vi "Read.vi"(4 "Error In":errorcluster, 5 "timeout ms (5000)":i32=5000, 7 "WebSocket Connection in":refnum<k5>) -> (0 "Error Out":errorcluster, 1 "Opcode":u8, 2 "Data":string, 3 "WebSocket Connection out":refnum<k5>)   [LabVIEW 2020, in "WebSockets.lvlib"]
doc: "Reads and decodes an incoming WebSockets message.\nWebSockets API 1.3.0.13\nSam Sharp - Intelligent Energy\nCopyright (c) 2015, Intelligent Energy"
uses:
  WebSockets.lvlib
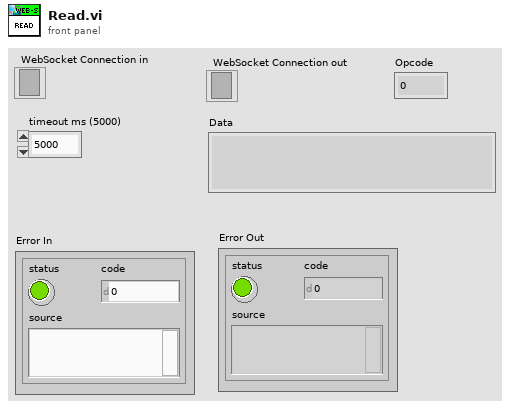
[diagram p1: front panel]
types:
  T1 = enum16{"big-endian, network order", "native, host order", "little-endian"}
  T2 = enum16{"Standard", "Buffered", "CRLF", "Immediate"}
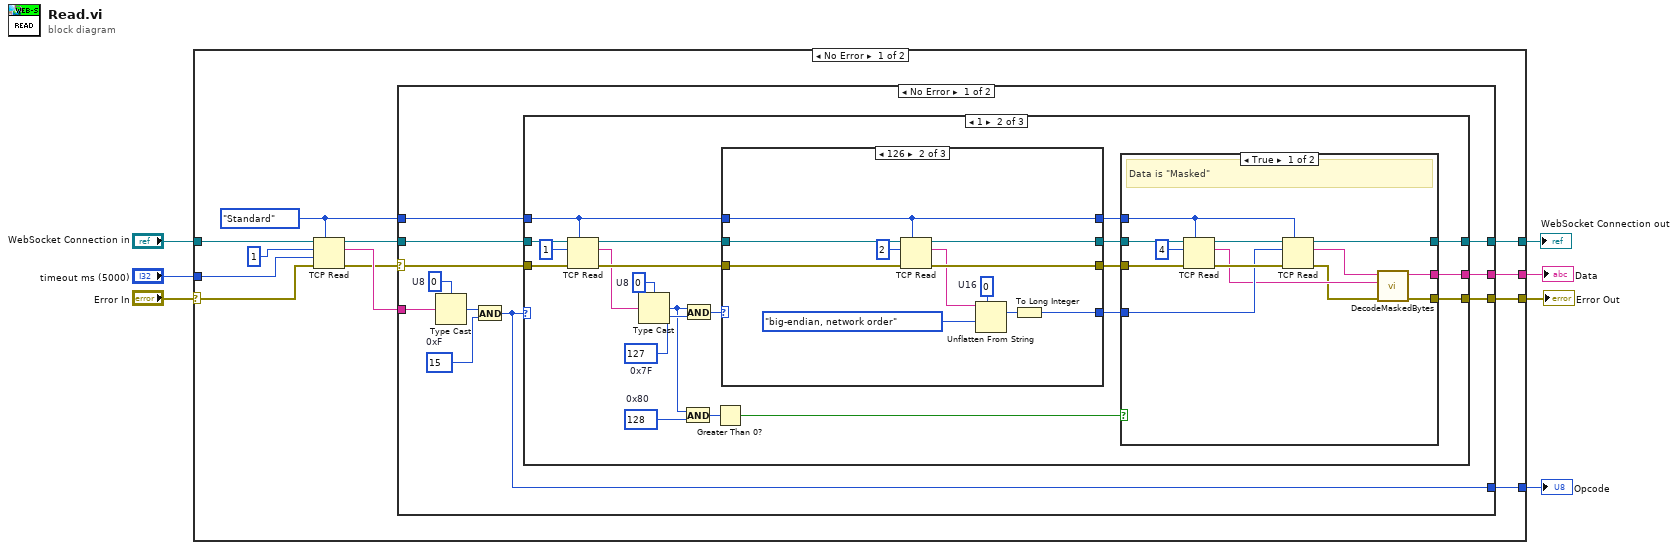
[diagram p0: block diagram]
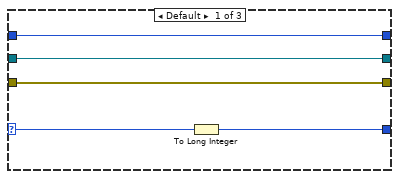
[diagram p3: hidden frame]
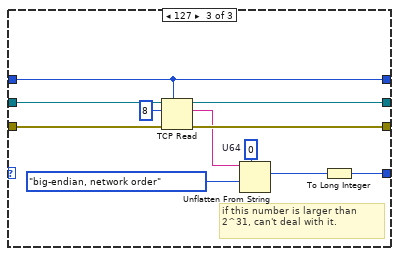
[diagram p4: hidden frame]
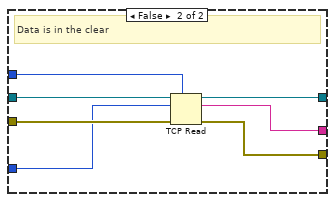
[diagram p5: hidden frame]
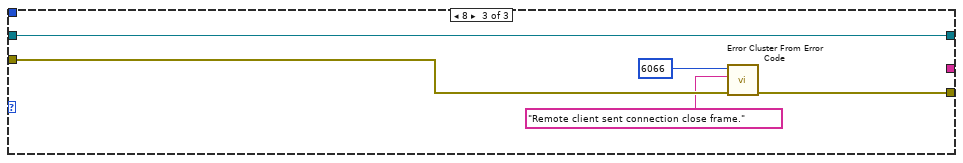
[diagram p6: hidden frame]
diagram:
  n1 = case shown="No Error" "Error In" {
    selector: "Error In" -> [w13 w109]
    tunnel: "WebSocket Connection in" -> [w19 w108]
    tunnel: [w14 w108] -> w6
    tunnel: [w12 _] -> w5
    tunnel: [w11 w109] -> w3
    tunnel: "timeout ms (5000)" -> [w10 _]
    tunnel: [w8 _] -> w1
    frame No Error {
      w15 = T2."Standard" ("mode (standard)")
      n2 = TCP Read(connection ID=w19, bytes to read=1, error in (no error)=w13, 7:w15, 9:w10) -> (connection ID out=w16:refnum<k5>, data out=w17:string, error out=w9:errorcluster)
      n3 = case shown="No Error" w9 {
        selector: w9 -> [w25 w106]
        tunnel: w17 -> [w24 _]
        tunnel: w16 -> [w30 w107]
        tunnel: w15 -> [w29 _]
        tunnel: [w28 w107] -> w14
        tunnel: [w27 _] -> w12
        tunnel: [w26 w106] -> w11
        tunnel: [w20 _] -> w8
        frame No Error {
          w21 = u8 15  # 0xF
          w23 = u8 0  # U8
          n4 = Type Cast(type=w23, x=w24) -> (*(type *) &x=w22:u8)
          n5 = And(x=w22, y=w21) -> (x .and. y?=w20:u8)
          n6 = case shown="1" w20 {
            tunnel: w30 -> [w32 w44 w105]
            tunnel: w29 -> [_ w42 _]
            tunnel: [w32 w53 w105] -> w28
            tunnel: [_ w46 _] -> w27
            tunnel: [w31 w45 w104] -> w26
            tunnel: w25 -> [w31 w40 w103]
            frame Default {
            }
            frame 1 {
              w36 = u8 128  # 0x80
              w37 = u8 0  # U8
              w52 = u8 127  # 0x7F
              n7 = TCP Read(connection ID=w44, bytes to read=1, error in (no error)=w40, 7:w42) -> (connection ID out=w43:refnum<k5>, data out=w38:string, error out=w39:errorcluster)  [unwired: 1 in]
              n8 = Type Cast(type=w37, x=w38) -> (*(type *) &x=w35:u8)
              n9 = And(x=w35, y=w36) -> (x .and. y?=w34:u8)
              n10 = And(x=w35, y=w52) -> (x .and. y?=w51:u8)
              n11 = Greater Than 0?(x=w34) -> (x > 0?=w33:bool)
              n12 = case shown="126" w51 {
                selector: w51 -> [w57 _ _]
                tunnel: w43 -> [w58 w69 w79]
                tunnel: [w58 w68 w78] -> w50
                tunnel: w42 -> [w55 w66 w74]
                tunnel: [w56 w59 w77] -> w47
                tunnel: [w55 w66 w74] -> w49
                tunnel: [w54 w65 w76] -> w48
                tunnel: w39 -> [w54 w64 w75]
                frame Default {
                  n13 = To Long Integer(number=w57) -> (32bit integer=w56:i32)
                }
                frame 126 {
                  w63 = u16 0  # U16
                  n14 = TCP Read(connection ID=w69, bytes to read=2, error in (no error)=w64, 7:w66) -> (connection ID out=w68:refnum<k5>, data out=w61:string, error out=w65:errorcluster)  [unwired: 1 in]
                  n15 = Unflatten From String(type=w63, binary string=w61, byte order (0:big-endian, network order)=T1."big-endian, network order") -> (value=w60:u16)  [unwired: 2 in, 2 out]
                  n16 = To Long Integer(number=w60) -> (32bit integer=w59:i32)
                }
                frame 127 {
                  w73 = u64 0  # U64
                  # "if this number is larger than\n2^31, can't deal with it."
                  n17 = TCP Read(connection ID=w79, bytes to read=8, error in (no error)=w75, 7:w74) -> (connection ID out=w78:refnum<k5>, data out=w72:string, error out=w76:errorcluster)  [unwired: 1 in]
                  n18 = Unflatten From String(type=w73, binary string=w72, byte order (0:big-endian, network order)=T1."big-endian, network order") -> (value=w71:u64)  [unwired: 2 in, 2 out]
                  n19 = To Long Integer(number=w71) -> (32bit integer=w77:i32)
                }
              }
              n20 = case shown="True" w33 {
                tunnel: [w93 w100] -> w53
                tunnel: w50 -> [w92 w99]
                tunnel: w49 -> [w90 w98]
                tunnel: w48 -> [w89 w97]
                tunnel: w47 -> [w86 w96]
                tunnel: [w83 w94] -> w46
                tunnel: [w81 w95] -> w45
                frame True {
                  # "Data is \"Masked\""
                  n21 = TCP Read(connection ID=w92, bytes to read=4, error in (no error)=w89, 7:w90) -> (connection ID out=w91:refnum<k5>, data out=w85:string, error out=w88:errorcluster)  [unwired: 1 in]
                  n22 = TCP Read(connection ID=w91, bytes to read=w86, error in (no error)=w88, 7:w90) -> (connection ID out=w93:refnum<k5>, data out=w84:string, error out=w82:errorcluster)  [unwired: 1 in]
                  n23 = call "DecodeMaskedBytes.vi"("error in (no error)"=w82, "Mask Bytes"=w85, "Encoded Data"=w84) -> ("error out"=w81:errorcluster, "Decoded Data"=w83:string)  [unwired: 3 in]
                }
                frame False {
                  # "Data is in the clear"
                  n24 = TCP Read(connection ID=w99, bytes to read=w96, error in (no error)=w97, 7:w98) -> (connection ID out=w100:refnum<k5>, data out=w94:string, error out=w95:errorcluster)  [unwired: 1 in]
                }
              }
            }
            frame 8 {
              n25 = call <vilib>:"Error Cluster From Error Code.vi"("error in (no error)"=w103, "error message (\"\")"="Remote client sent connection close frame." ("error message (\"\")"), "error code (0)"=6066) -> ("error out"=w104:errorcluster)  [unwired: 6 in]
            }
          }
        }
        frame Error {
        }
      }
    }
    frame Error {
    }
  }
  "WebSocket Connection out" <- w6
  "Data" <- w5
  "Error Out" <- w3
  "Opcode" <- w1
